vi "TunnelFactory.vi"(8 "error in":errorcluster, 11 "reference":refnum<vi>) -> (0 "error out":errorcluster, 3 "Tunnel out":refnum<class "Tunnel.lvclass">)   [LabVIEW 2014, in "Raspberry Pi Compatible Compiler for LabVIEW.lvlib" / "Tunnel.lvclass"]
uses:
  Tunnel.lvclass
  LoopTunnel/LoopTunnel.lvclass
  RightShiftRegister/RightShiftRegister.lvclass
  LeftShiftRegister/LeftShiftRegister.lvclass
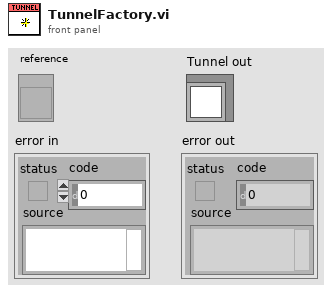
[diagram p1: front panel]
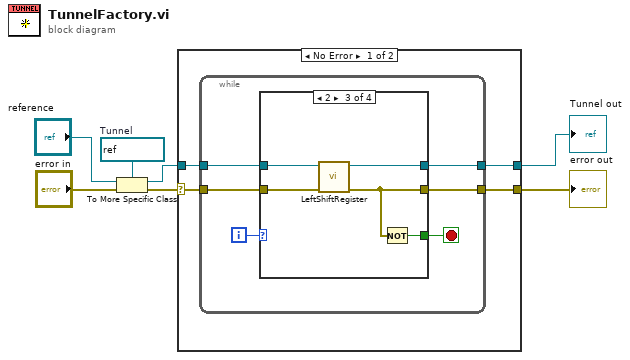
[diagram p0: block diagram]
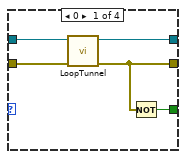
[diagram p2: hidden frame]
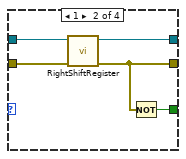
[diagram p3: hidden frame]
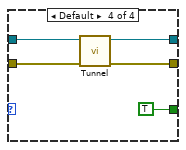
[diagram p4: hidden frame]
diagram:
  w5 = refnum<vi> refnum  # Tunnel
  n1 = To More Specific Class(target class=w5, reference="reference", error in="error in") -> (specific class reference=w2:refnum<vi>, error out=w3:errorcluster)
  n2 = case shown="No Error" w3 {
    selector: w3 -> [w11 w38]
    tunnel: [w9 _] -> w7
    tunnel: [w8 w38] -> w6
    tunnel: w2 -> [w10 _]
    frame No Error {
      n3 = while {
        tunnel: w11 -> [w16]
        tunnel: [w15] -> w8
        tunnel: [w14] -> w9
        tunnel: w10 -> [w12]
        i -> [w17]
        stop <- w13 stop-if-true
        n4 = case shown="2" w17 {
          tunnel: w16 -> [w18 w23 w28 w34]
          tunnel: [w19 w24 w29 w33] -> w15
          tunnel: [w20 w25 w30 w36] -> w14
          tunnel: [w22 w27 w32 TRUE] -> w13
          tunnel: w12 -> [w21 w26 w31 w35]
          frame 0 {
            n5 = call "LoopTunnel.vi"("error in"=w18, "reference"=w21) -> ("error out"=w19:errorcluster, "LoopTunnel out"=w20:refnum<class "LoopTunnel.lvclass">)  [unwired: 8 in]
            n6 = Not(x=w19) -> (.not. x?=w22:bool)
          }
          frame 1 {
            n7 = call "RightShiftRegister.vi"("error in"=w23, "reference"=w26) -> ("error out"=w24:errorcluster, "ShiftRegister out"=w25:refnum<class "RightShiftRegister.lvclass">)  [unwired: 8 in]
            n8 = Not(x=w24) -> (.not. x?=w27:bool)
          }
          frame 2 {
            n9 = call "LeftShiftRegister.vi"("error in"=w28, "reference"=w31) -> ("error out"=w29:errorcluster, "ShiftRegister out"=w30:refnum<class "LeftShiftRegister.lvclass">)  [unwired: 8 in]
            n10 = Not(x=w29) -> (.not. x?=w32:bool)
          }
          frame Default {
            n11 = call "Tunnel.vi"("error in"=w34, "reference"=w35) -> ("error out"=w33:errorcluster, "Tunnel out"=w36:refnum<class "Tunnel.lvclass">)  [unwired: 8 in]
          }
        }
      }
    }
    frame Error {
    }
  }
  "error out" <- w6
  "Tunnel out" <- w7
